vi "sick_ground filter.vi"() -> ()   [LabVIEW 2015]
uses:
  <vilib>/Analysis/6fits.llb/Curve Fitting Criteria.ctl
  G_SEN.vi
  <vilib>/Analysis/polynomials.llb/1D Polynomial Evaluation (DBL).vi
  <vilib>/Analysis/NI_AALPro.lvlib
panel:
  out "sick_rear":dbl[][](array[numeric])
  out "abs(x)":dbl[](array[numeric])
  out "Polynomial Coefficients":dbl[](array[numeric])
  in  "z_thresh":dbl=0.25 format="%#_13g"
  out "I":dbl[](array[numeric])
  out "XY Graph 2":cluster{"Y":dbl[], "Y":dbl[]}[](graph)
  in  "transposed array 2":dbl[][](array[numeric])
  in  "thresh":dbl=5.0 format="%#_13g"
  out "XY Graph":cluster{"Y":dbl[], "Y":dbl[]}[](graph)
  in  "diff":i32=1
  out "X":dbl[](array[numeric])
  out "Y":dbl[](array[numeric])
  out "Z":dbl[](array[numeric])
  out "obs":i32[](array[numeric])
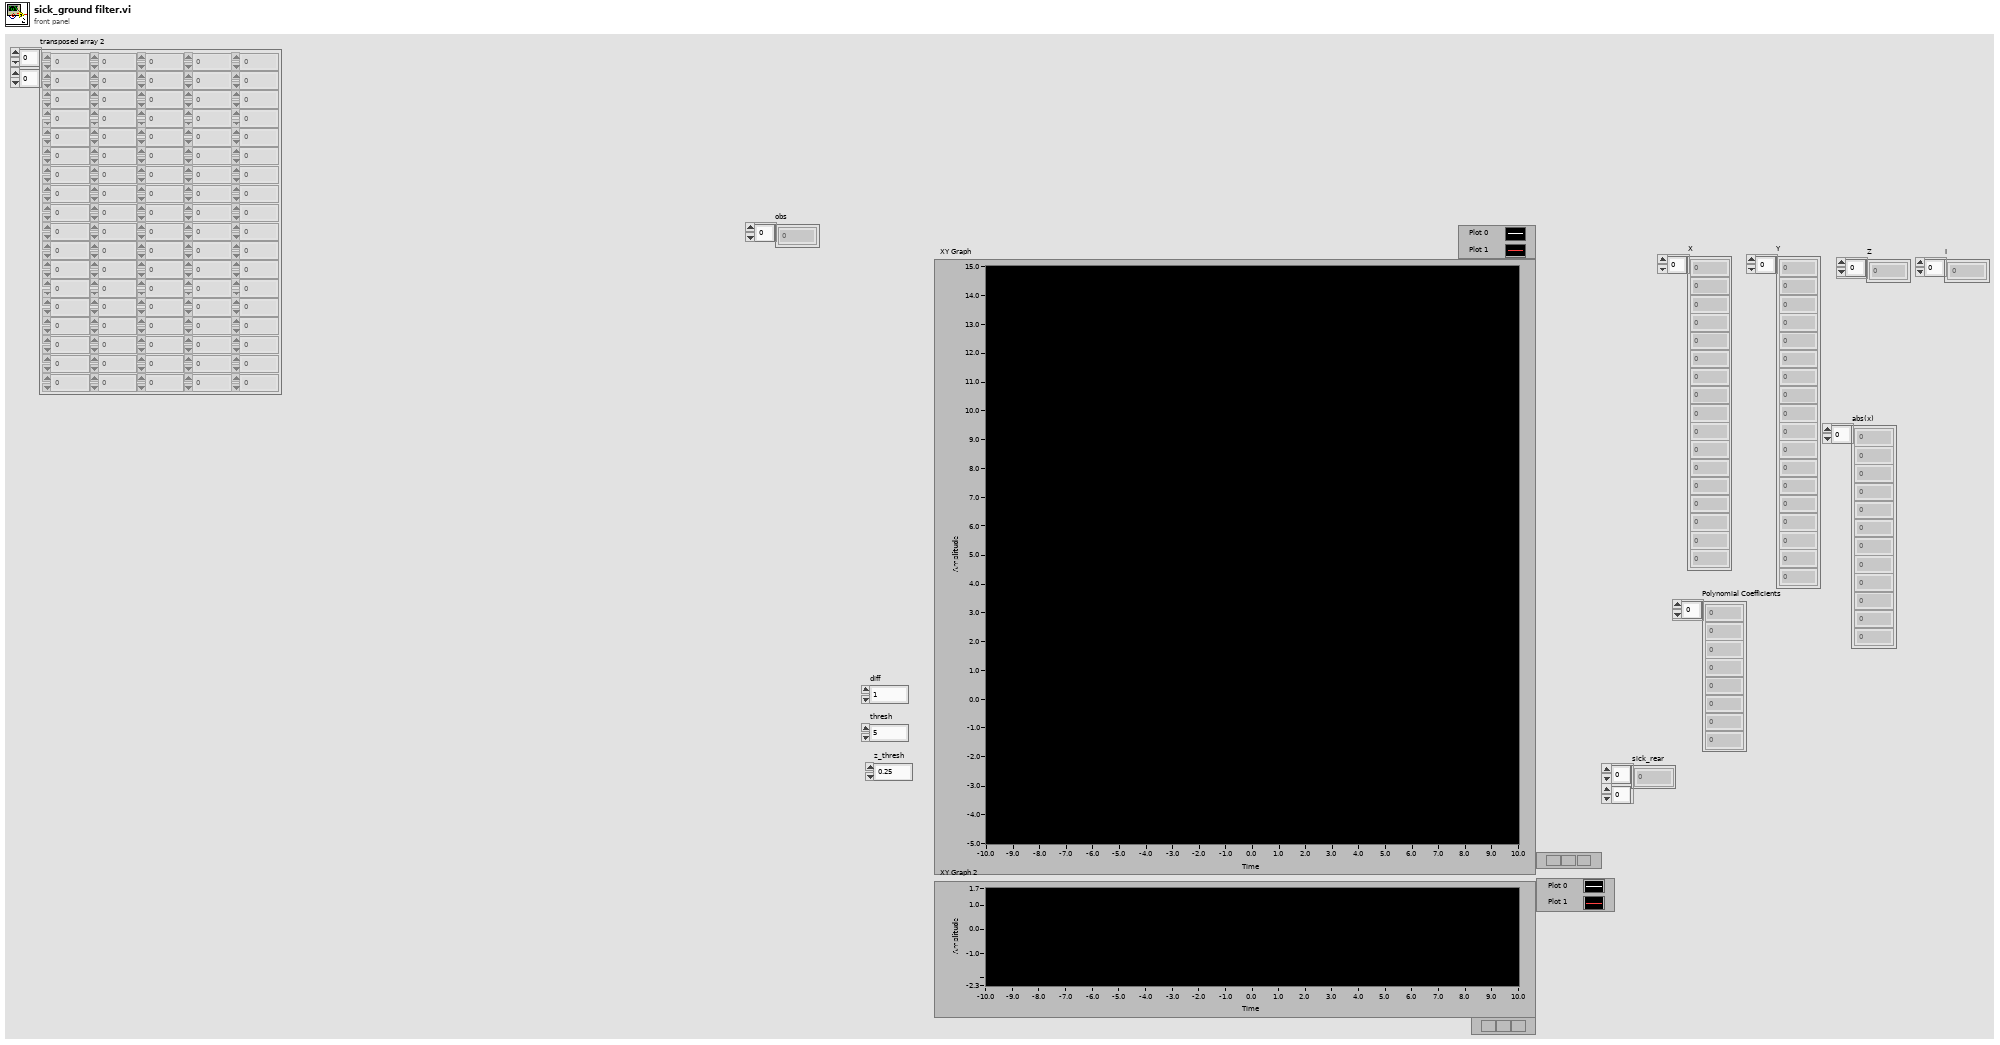
[diagram p1: front panel]
types:
  T1 = typedef "NI_AALPro.lvlib/Curve Fitting Criteria.ctl" = u16
  T2 = cluster{i32, "Rotational position":dbl, "Rotational position":dbl, "Rotational position":dbl, "element":dbl}[]
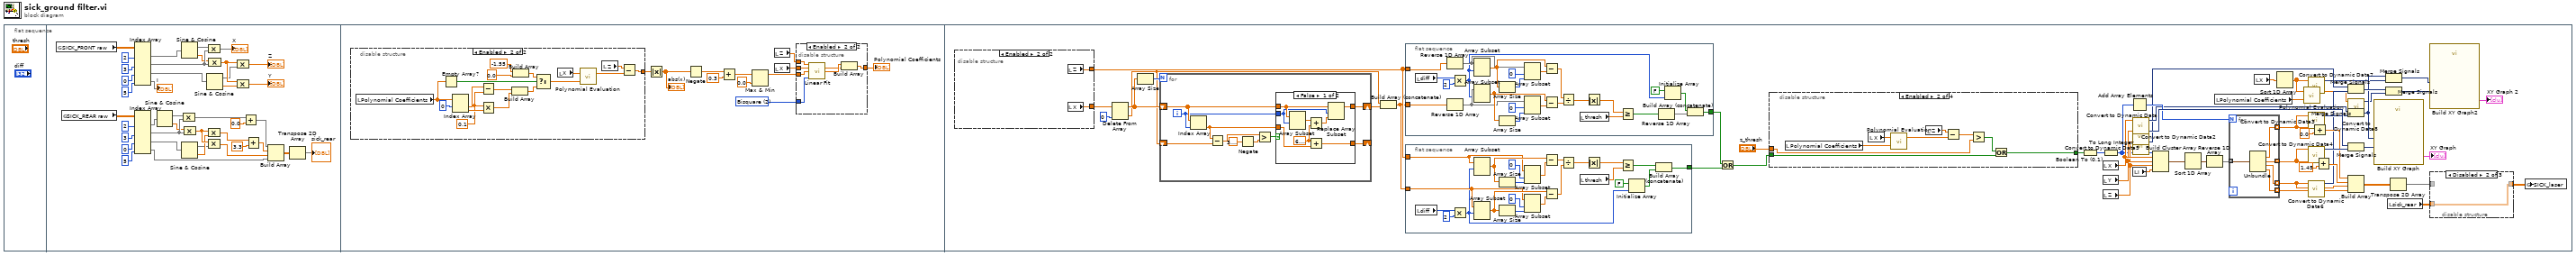
[diagram p0: block diagram]
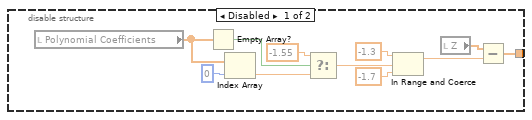
[diagram p2: hidden frame]
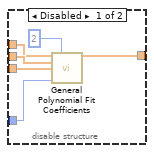
[diagram p3: hidden frame]
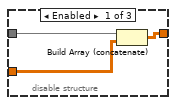
[diagram p4: hidden frame]
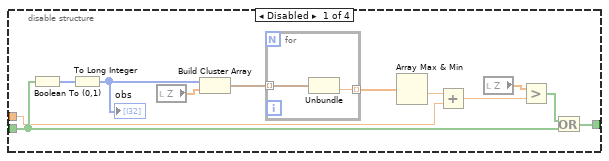
[diagram p6: hidden frame]
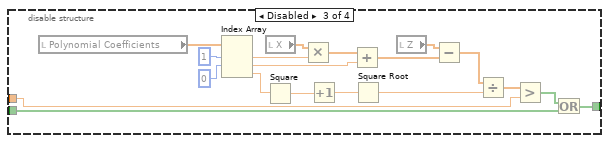
[diagram p7: hidden frame]
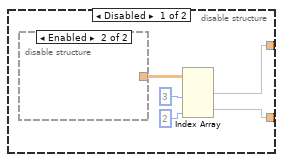
[diagram p9: hidden frame]
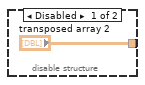
[diagram p10: hidden frame]
diagram:
  n1 = flat-sequence {
    frame #0 {
    }
    frame #1 {
      n2 = global read "G_SEN.vi" "SICK_FRONT raw"() -> (w31:dbl[][])
      n3 = global read "G_SEN.vi" "SICK_REAR raw"() -> (w16:dbl[][])
      n4 = Index Array(array=w31, index (col) #1=2 ("disabled index (col)"), index (col) #2=3 ("index (col)"), index (col) #3=0 ("index (col)"), index (col) #4=5 ("index (col)")) -> (element #1=w32:dbl[], element #2=w35:dbl[], element #3=w37:dbl[], element #4=→"I":dbl[])  [unwired: 4 in]
      n5 = Index Array(array=w16, index (col) #1=2 ("disabled index (col)"), index (col) #2=3 ("index (col)"), index (col) #3=0 ("index (col)"), index (col) #4=5 ("index (col)")) -> (element #1=w17:dbl[], element #2=w20:dbl[], element #3=w21:dbl[], element #4=w3:dbl[])  [unwired: 4 in]
      n6 = Sine & Cosine(0:w17) -> (1:w18:dbl[], 2:w19:dbl[])
      n7 = Sine & Cosine(0:w32) -> (1:w33:dbl[], 2:w34:dbl[])
      n8 = Sine & Cosine(0:w21) -> (1:w11:dbl[], 2:w22:dbl[])
      n9 = Compound Arithmetic op=MULTIPLY(w18, w20) -> (w10:dbl[])
      n10 = Compound Arithmetic op=MULTIPLY(w19, w20) -> (w23:dbl[])
      n11 = Sine & Cosine(0:w37) -> (1:w25:dbl[], 2:w38:dbl[])
      n12 = Compound Arithmetic op=MULTIPLY(w33, w35) -> (→"X":dbl[])
      n13 = Compound Arithmetic op=MULTIPLY(w23, w22) -> (w8:dbl[])
      n14 = Compound Arithmetic op=MULTIPLY(w23, w11) -> (w4:dbl[])
      n15 = Compound Arithmetic op=MULTIPLY(w34, w35) -> (w40:dbl[])
      n16 = Compound Arithmetic op=MULTIPLY(w40, w25) -> (→"Z":dbl[])
      n17 = Compound Arithmetic op=MULTIPLY(w40, w38) -> (→"Y":dbl[])
      n18 = Add(x=w10, y=0.0 ("x_off")) -> (x+y=w6:dbl[])
      n19 = Add(x=w8, y=3.3 ("y_off 2")) -> (x+y=w5:dbl[])
      n20 = Build Array(w6, w5, w4, w3) -> (w2:dbl[][])
      n21 = Transpose 2D Array(2D array=w2) -> (transposed array=→"sick_rear":dbl[][])
    }
    frame #2 {
      w41 = T1 2 items=["Least Square", "Least Absolute Residual", "Bisquare"] ("method")
      n22 = disable-structure shown="Enabled" {
        disable-tunnel: [w61 w71] -> w49
        frame Disabled {
          n23 = local read "Polynomial Coefficients"() -> (w58:dbl[])
          n24 = Empty Array?(array=w58) -> (empty?=w60:bool)
          n25 = Index Array(array=w58, index=0) -> (element=w57:dbl)
          n26 = Select(t=-1.55, s=w60, f=w57) -> (s? t:f=w55:dbl)
          n27 = In Range and Coerce(upper limit=-1.3, x=w55, lower limit=-1.7) -> (coerced(x)=w54:dbl)  [unwired: 1 out]
          n28 = local read "Z"() -> (w62:dbl[])
          n29 = Subtract(x=w62, y=w54) -> (x-y=w61:dbl[])
        }
        frame Enabled {
          w66 = 0.1
          n30 = local read "Polynomial Coefficients"() -> (w70:dbl[])
          n31 = Empty Array?(array=w70) -> (empty?=w77:bool)
          n32 = Index Array(array=w70, index #1=0 ("index")) -> (element #1=w68:dbl, element #2=w67:dbl)  [unwired: 1 in]
          n33 = Subtract(x=w68, y=w66) -> (x-y=w65:dbl)
          n34 = Multiply(x=w66, y=w67) -> (x*y=w64:dbl)
          n35 = Build Array(w65, w64) -> (w63:dbl[])
          n36 = Build Array(-1.55, 0.0 ("element")) -> (w78:dbl[])
          n37 = Select(t=w78, s=w77, f=w63) -> (s? t:f=w79:dbl[])
          n38 = local read "X"() -> (w72:dbl[])
          n39 = call-poly <vilib>:"Polynomial Evaluation.vi"("P(x)"=w79, "A"=w72) -> ("P(A)"=w74:dbl[])  [unwired: 1 out]
          n40 = local read "Z"() -> (w73:dbl[])
          n41 = Subtract(x=w73, y=w74) -> (x-y=w71:dbl[])
        }
      }
      n42 = Absolute Value(x=w49) -> (abs(x)=w48:dbl[])
      "abs(x)" <- w48
      n43 = Negate(x=w48) -> (-x=w47:dbl[])
      n44 = Add(x=w47, y=0.3) -> (x+y=w46:dbl[])
      n45 = Max & Min(x=w46, y=0.0) -> (max(x,y)=w43:dbl[])  [unwired: 1 out]
      n46 = local read "Z"() -> (w50:dbl[])
      n47 = local read "X"() -> (w51:dbl[])
      n48 = disable-structure shown="Enabled" {
        disable-tunnel: w51 -> [w85 w91]
        disable-tunnel: w50 -> [w84 w92]
        disable-tunnel: w43 -> [w82 w90]
        disable-tunnel: [w81 w86] -> w42
        disable-tunnel: w41 -> [w80 w89]
        frame Disabled {
          n49 = call <vilib>:"General Polynomial Fit Coefficients.vi"("Y"=w84, "polynomial order"=2, "X"=w85, "Weight"=w82, "method"=w80) -> ("Polynomial Coefficients"=w81:dbl[])  [unwired: 9 in, 1 out]
        }
        frame Enabled {
          n50 = call <vilib>:"Linear Fit.vi"("Y"=w92, "X"=w91, "Weight"=w90, "method"=w89) -> ("slope"=w87:dbl, "intercept"=w88:dbl)  [unwired: 7 in, 3 out]
          n51 = Build Array(w88, w87) -> (w86:dbl[])
        }
      }
      "Polynomial Coefficients" <- w42
    }
    frame #3 {
      n52 = disable-structure shown="Enabled" {
        disable-tunnel: [w199 w201] -> w146
        disable-tunnel: [w196 w202] -> w123
        frame Disabled {
          n53 = disable-structure shown="Enabled" {
            disable-tunnel: ["transposed array 2" _] -> w198
            frame Disabled {
            }
            frame Enabled {
            }
          }
          n54 = Index Array(array=w198, index (col) #1=3 ("disabled index (col)"), index (col) #2=2 ("disabled index (col)")) -> (element #1=w199:dbl[], element #2=w196:dbl[])  [unwired: 2 in]
        }
        frame Enabled {
          n55 = local read "Z"() -> (w201:dbl[])
          n56 = local read "X"() -> (w202:dbl[])
        }
      }
      n57 = Delete From Array(array=w123, index=0) -> (deleted portion=w124:dbl, array with subset deleted=w126:dbl[])  [unwired: 1 in]
      n58 = Array Size(array=w126) -> (size(s)=w127:i32)
      n59 = for {
        N: w127 -> [_]
        shift-right: [w259] -> w125
        shift-left: w126 -> [w258]
        shift-right: [w257] -> _
        shift-left: w124 -> [w254]
        i -> [w256]
        n60 = Index Array(array=w258, index=w256) -> (element=w255:dbl)
        n61 = Subtract(x=w255, y=w254) -> (x-y=w251:dbl)
        n62 = Negate(x=3.141592653589793) -> (-x=w252:dbl)
        n63 = Greater?(x=w251, y=w252) -> (0:w250:bool)
        n64 = case shown="False" w250 {
          tunnel: [w263 w269] -> w259
          tunnel: w258 -> [w266 w269]
          tunnel: [w260 w268] -> w257
          tunnel: w255 -> [w261 w268]
          tunnel: w256 -> [w265 _]
          frame False {
            w262 = 6.283185307179586
            n65 = Array Subset(array=w266, index=w265) -> (w267:dbl[])  [unwired: 1 in]
            n66 = Add(x=w267, y=w262) -> (x+y=w264:dbl[])
            n67 = Add(x=w262, y=w261) -> (x+y=w260:dbl)
            n68 = Replace Array Subset(array=w266, new element=w264, index=w265) -> (w263:dbl[])
          }
          frame True {
          }
        }
      }
      n69 = Build Array (concatenate)(w124, w125) -> (w122:dbl[])
      n70 = flat-sequence {
        tunnel: w146 -> [w211]
        tunnel: w122 -> [w209]
        tunnel: [w214] -> w121
        frame #0 {
          n71 = local read "diff"() -> (w212:i32)
          n72 = Reverse 1D Array(array=w211) -> (reversed array=w210:dbl[])
          n73 = Reverse 1D Array(array=w209) -> (reversed array=w208:dbl[])
          n74 = Multiply(x=w212, y=2) -> (x*y=w204:i32)
          n75 = Array Subset(array=w210, index=w204) -> (w223:dbl[])  [unwired: 1 in]
          n76 = Array Subset(array=w208, index=w204) -> (w219:dbl[])  [unwired: 1 in]
          n77 = Array Size(array=w223) -> (size(s)=w222:i32)
          n78 = Array Size(array=w219) -> (size(s)=w218:i32)
          n79 = Array Subset(array=w210, index=0, length=w222) -> (w220:dbl[])
          n80 = Array Subset(array=w208, index=0, length=w218) -> (w216:dbl[])
          n81 = Subtract(x=w223, y=w220) -> (x-y=w226:dbl[])
          n82 = Subtract(x=w219, y=w216) -> (x-y=w227:dbl[])
          n83 = Divide(x=w226, y=w227) -> (x/y=w225:dbl[])
          n84 = local read "thresh"() -> (w203:dbl)
          n85 = Absolute Value(x=w225) -> (abs(x)=w224:dbl[])
          n86 = Greater Or Equal?(x=w224, y=w203) -> (x >= y?=w207:bool[])
          n87 = Reverse 1D Array(array=w207) -> (reversed array=w206:bool[])
          n88 = Initialize Array(FALSE, w204) -> (w205:bool[])
          n89 = Build Array (concatenate)(w205, w206) -> (w214:bool[])
        }
      }
      n90 = flat-sequence {
        tunnel: w146 -> [w245]
        tunnel: w122 -> [w239]
        tunnel: [w235] -> w120
        frame #0 {
          n91 = local read "diff"() -> (w233:i32)
          n92 = Multiply(x=w233, y=2) -> (x*y=w230:i32)
          n93 = Array Subset(array=w245, index=w230) -> (w246:dbl[])  [unwired: 1 in]
          n94 = Array Subset(array=w239, index=w230) -> (w241:dbl[])  [unwired: 1 in]
          n95 = Array Size(array=w246) -> (size(s)=w244:i32)
          n96 = Array Size(array=w241) -> (size(s)=w240:i32)
          n97 = Array Subset(array=w245, index=0, length=w244) -> (w242:dbl[])
          n98 = Array Subset(array=w239, index=0, length=w240) -> (w237:dbl[])
          n99 = Subtract(x=w246, y=w242) -> (x-y=w248:dbl[])
          n100 = Subtract(x=w241, y=w237) -> (x-y=w249:dbl[])
          n101 = Divide(x=w248, y=w249) -> (x/y=w247:dbl[])
          n102 = local read "thresh"() -> (w229:dbl)
          n103 = Absolute Value(x=w247) -> (abs(x)=w228:dbl[])
          n104 = Greater Or Equal?(x=w228, y=w229) -> (x >= y?=w231:bool[])
          n105 = Initialize Array(FALSE, w230) -> (w232:bool[])
          n106 = Build Array (concatenate)(w231, w232) -> (w235:bool[])
        }
      }
      n107 = Or(x=w121, y=w120) -> (x .or. y?=w105:bool[])
      n108 = disable-structure shown="Enabled" {
        disable-tunnel: [w154 w173 w178 w194] -> w106
        disable-tunnel: w105 -> [w153 w174 w179 w194]
        disable-tunnel: "z_thresh" -> [w152 w166 w175 _]
        frame Disabled {
          n109 = Boolean To (0,1)(Boolean=w153) -> (0, 1=w163:i16[])
          n110 = To Long Integer(number=w163) -> (32bit integer=w159:i32[])
          "obs" <- w159
          n111 = local read "Z"() -> (w158:dbl[])
          n112 = Build Cluster Array(w159, w158) -> (w157:cluster{i32, "Rotational position":dbl}[])
          n113 = for {
            tunnel: w157 -> [w165] mode=indexing
            tunnel: [w164] -> w156 mode=indexing
            n114 = Unbundle(w165) -> ("Rotational position"=w164:dbl)  [unwired: 1 out]
          }
          n115 = Array Max & Min(array=w156) -> (min value=w162:dbl)  [unwired: 3 out]
          n116 = Add(x=w162, y=w152) -> (x+y=w161:dbl)
          n117 = local read "Z"() -> (w160:dbl[])
          n118 = Greater?(x=w160, y=w161) -> (0:w155:bool[])
          n119 = Or(x=w155, y=w153) -> (x .or. y?=w154:bool[])
        }
        frame Enabled {
          n120 = local read "Polynomial Coefficients"() -> (w171:dbl[])
          n121 = local read "X"() -> (w170:dbl[])
          n122 = call-poly <vilib>:"Polynomial Evaluation.vi"("P(x)"=w171, "A"=w170) -> ("P(A)"=w168:dbl[])  [unwired: 1 out]
          n123 = local read "Z"() -> (w169:dbl[])
          n124 = Subtract(x=w169, y=w168) -> (x-y=w167:dbl[])
          n125 = Greater?(x=w167, y=w166) -> (0:w172:bool[])
          n126 = Or(x=w172, y=w174) -> (x .or. y?=w173:bool[])
        }
        frame Disabled {
          n127 = local read "Polynomial Coefficients"() -> (w193:dbl[])
          n128 = Index Array(array=w193, index #1=1 ("index"), index #2=0 ("index")) -> (element #1=w190:dbl, element #2=w187:dbl, element #3=w184:dbl)  [unwired: 1 in]
          n129 = Square(x=w184) -> (x^2=w183:dbl)
          n130 = local read "X"() -> (w191:dbl[])
          n131 = Multiply(x=w191, y=w190) -> (x*y=w189:dbl[])
          n132 = Increment(x=w183) -> (x+1=w182:dbl)
          n133 = Add(x=w189, y=w187) -> (x+y=w186:dbl[])
          n134 = Square Root(x=w182) -> (sqrt(x)=w181:dbl)
          n135 = local read "Z"() -> (w185:dbl[])
          n136 = Subtract(x=w185, y=w186) -> (x-y=w176:dbl[])
          n137 = Divide(x=w176, y=w181) -> (x/y=w180:dbl[])
          n138 = Greater?(x=w180, y=w175) -> (0:w177:bool[])
          n139 = Or(x=w177, y=w179) -> (x .or. y?=w178:bool[])
        }
        frame Disabled {
        }
      }
      n140 = Boolean To (0,1)(Boolean=w106) -> (0, 1=w108:i16[])
      n141 = To Long Integer(number=w108) -> (32bit integer=w107:i32[])
      n142 = local read "X"() -> (w113:dbl[])
      n143 = local read "Y"() -> (w112:dbl[])
      n144 = local read "Z"() -> (w111:dbl[])
      n145 = Add Array Elements(numeric array=w107) -> (sum=w140:i32)
      n146 = call "Convert to Dynamic Data"("Array"=w113) -> ("Dynamic Data Type"=w118:dynamicdata)  [unwired: 3 in]
      n147 = call "Convert to Dynamic Data2"("Array"=w112) -> ("Dynamic Data Type"=w143:dynamicdata)  [unwired: 3 in]
      n148 = call "Convert to Dynamic Data5"("Array"=w111) -> ("Dynamic Data Type"=w117:dynamicdata)  [unwired: 3 in]
      n149 = local read "I"() -> (w110:dbl[])
      n150 = Build Cluster Array(w107, w113, w112, w111, w110) -> (w142:T2)
      n151 = Sort 1D Array(array=w142) -> (sorted array=w141:T2)
      n152 = Reverse 1D Array(array=w141) -> (reversed array=w139:T2)
      n153 = local read "Polynomial Coefficients"() -> (w104:dbl[])
      n154 = for {
        N: w140 -> [_]
        tunnel: w139 -> [w274] mode=indexing
        tunnel: [w273] -> w135 mode=indexing
        tunnel: [w272] -> w131 mode=indexing
        tunnel: [w271] -> w109 mode=indexing
        tunnel: [w270] -> w129 mode=indexing
        n155 = Unbundle(w274) -> ("Rotational position"=w273:dbl, "Rotational position"=w272:dbl, "Rotational position"=w271:dbl, "element"=w270:dbl)  [unwired: 1 out]
      }
      n156 = local read "X"() -> (w98:dbl[])
      n157 = Sort 1D Array(array=w98) -> (sorted array=w97:dbl[])
      n158 = call-poly <vilib>:"Polynomial Evaluation.vi"("P(x)"=w104, "A"=w97) -> ("P(A)"=w100:dbl[])  [unwired: 1 out]
      n159 = call "Convert to Dynamic Data7"("Array"=w97) -> ("Dynamic Data Type"=w102:dynamicdata)  [unwired: 3 in]
      n160 = call "Convert to Dynamic Data3"("Array"=w135) -> ("Dynamic Data Type"=w138:dynamicdata)  [unwired: 3 in]
      n161 = call "Convert to Dynamic Data4"("Array"=w131) -> ("Dynamic Data Type"=w137:dynamicdata)  [unwired: 3 in]
      n162 = call "Convert to Dynamic Data6"("Array"=w109) -> ("Dynamic Data Type"=w116:dynamicdata)  [unwired: 3 in]
      n163 = Add(x=w135, y=0.0) -> (x+y=w133:dbl[])
      n164 = Add(x=w131, y=1.45) -> (x+y=w130:dbl[])
      n165 = Merge Signals(w117, w116) -> (w115:dynamicdata)
      n166 = call "Convert to Dynamic Data8"("Array"=w100) -> ("Dynamic Data Type"=w99:dynamicdata)  [unwired: 3 in]
      n167 = Merge Signals(w118, w138) -> (w114:dynamicdata)
      n168 = Merge Signals(w143, w137) -> (w145:dynamicdata)
      n169 = Build Array(w133, w130, w109, w129) -> (w136:dbl[][])
      n170 = call "Build XY Graph"("Y Input"=w145, "X Input"=w114) -> ("XY Graph"=→"XY Graph":cluster{"X":dbl[], "Y":dbl[]}[])  [unwired: 8 in, 1 out]
      n171 = Merge Signals(w114, w102) -> (w103:dynamicdata)
      n172 = Merge Signals(w115, w99) -> (w101:dynamicdata)
      n173 = local read "sick_rear"() -> (w93:dbl[][])
      n174 = Transpose 2D Array(2D array=w136) -> (transposed array=w95:dbl[][])
      n175 = call "Build XY Graph2"("Y Input"=w101, "X Input"=w103) -> ("XY Graph"=→"XY Graph 2":cluster{"X":dbl[], "Y":dbl[]}[])  [unwired: 8 in, 1 out]
      n176 = disable-structure shown="Disabled" {
        disable-tunnel: w95 -> [w149 _ w151]
        disable-tunnel: [w148 w150 w151] -> w94
        disable-tunnel: w93 -> [w147 w150 _]
        frame Enabled {
          n177 = Build Array (concatenate)(w149, w147) -> (w148:dbl[][])
        }
        frame Disabled {
        }
        frame Disabled {
        }
      }
      n178 = global write "G_SEN.vi" "SICK_laser"(w94) -> ()
    }
  }
